vi "Test Bench v12.vi"() -> ()   [LabVIEW 2022 SP3]
uses:
  WhiteNoise.ctl
  <vilib>/Utility/error.llb/DialogType.ctl
  <vilib>/DAQmx/read.llb/DAQmx Read (Analog 1D DBL 1Chan NSamp).vi
  <vilib>/DAQmx/write.llb/DAQmx Write (Analog 2D DBL NChan NSamp).vi
  <vilib>/DAQmx/create/channels.llb/DAQmx Create Channel (AI-Acceleration-Accelerometer).vi
  <vilib>/DAQmx/create/channels.llb/DAQmx Create Channel (AO-Voltage-Basic).vi
  <vilib>/DAQmx/configure/timing.llb/DAQmx Timing (Sample Clock).vi
  <vilib>/DAQmx/miscellaneous.llb/DAQmx Fill In Error Info.vi
  <resource>/objmgr/daqmx.rc
  <vilib>/measure/NI_MABase.lvlib
  <vilib>/DAQmx/configure/task.llb/DAQmx Configure Logging (TDMS).vi
  <vilib>/Waveform/WDTOps.llb/WDT Get Waveform Time Array DBL.vi
panel:
  in  "Folder to save file to":path=path "C:/Users/LAV-UFSC/Documents/LAV-TCC/Dados-Experimentos/Dados-Bancada-LABVIEW"
  in  "Log Raw\nData":bool
  in  "Accel. 2":bool
  in  "Start\nReading":bool=TRUE
  out "New file path":path
  in  "Signal Output Control":enum32{"White Noise", "Harmonic"}(tab)
  in  "White Noise\nParameters":T2={"Seed"=0.0, "Standard Deviation"=0.2, "Reset"=FALSE, "Iterator"=1.0, "Seed"=-1, "Stop 4"=FALSE, "Lower Cut-Off"=5.0, "Upper Cut-Off"=350.0} {"Upper Cut-Off" min=5.0 max=350.0 step=10.0; "Lower Cut-Off" min=5.0 max=350.0 step=10.0; "Standard Deviation" min=0.001 max=1.5 step=0.05 format="%0.2p"}
  in  "Hamonic\nParameters":T3={"Waveform Type"=0, "Frequency"=10.0, "Amplitude"=0.25, "Stop 4"=FALSE} {"Frequency" min=5.0 max=350.0 step=10.0 format="%0.2p"; "Waveform Type" items=["Sine Wave", "Triangle Wave", "Square Wave", "Sawtooth Wave"]; "Amplitude" min=0.001 max=0.3 step=0.05 format="%0.2p"}
  in  "Start\nOutput":bool=TRUE
  # "Filter"
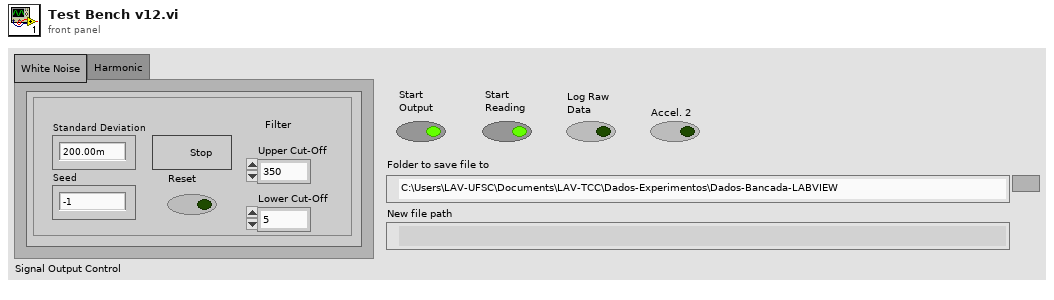
[diagram p1: front panel]
types:
  T1 = typedef "WhiteNoise.ctl" = dbl
  T2 = cluster{"Seed":T1, "Standard Deviation":dbl, "Reset":bool, "Iterator":dbl, "Seed":i8, "Stop 4":bool, "Lower Cut-Off":dbl, "Upper Cut-Off":dbl}
  T3 = cluster{"Waveform Type":u16, "Frequency":dbl, "Amplitude":dbl, "Stop 4":bool}
  T4 = typedef "DialogType.ctl" = u16
  T5 = enum16{"open", "open or create", "create or replace", "create", "open (read-only)"}
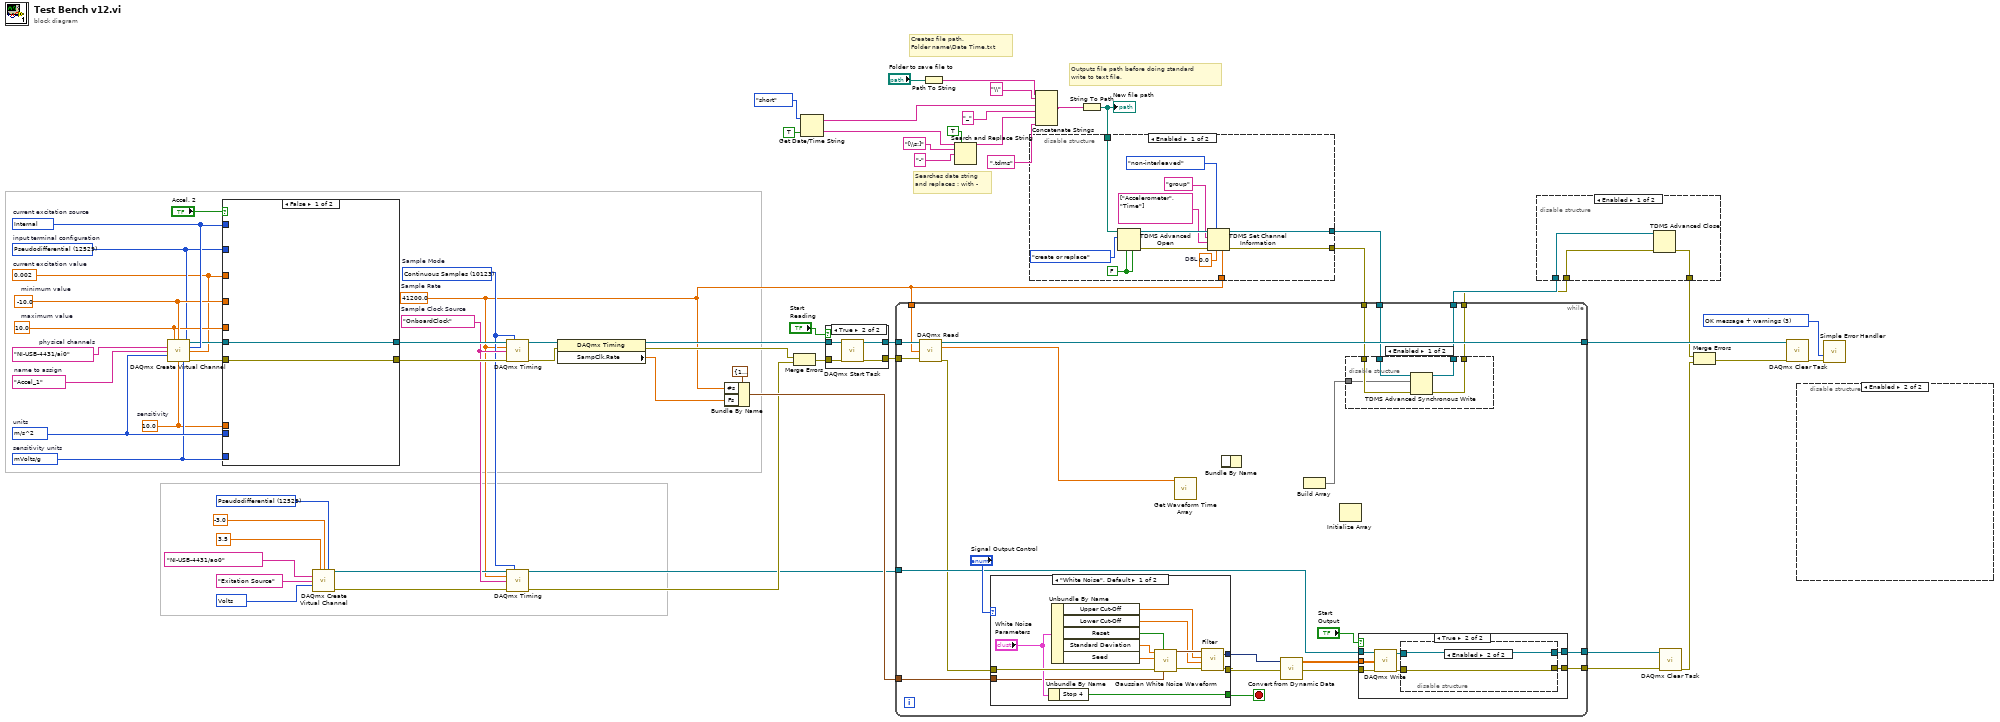
[diagram p0: block diagram]
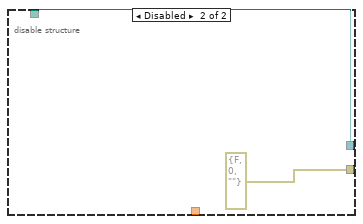
[diagram p2: hidden frame]
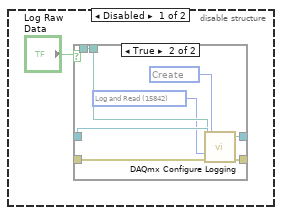
[diagram p4: hidden frame]
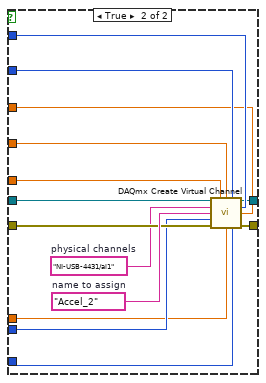
[diagram p6: hidden frame]
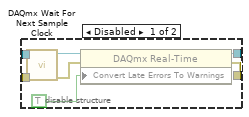
[diagram p10: hidden frame]
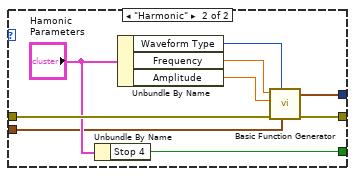
[diagram p11: hidden frame]
diagram:
  w40 = T4 3 items=["no dialog", "OK message", "continue or stop message", "OK message + warnings", "continue/stop + warnings"] ("type of dialog (OK msg:1)")
  w53 = 12529 items=["Default"=-1, "RSE"=10083, "Differential"=10106, "Pseudodifferential"=12529] ("output terminal configuration")
  w51 = 10348 items=["Volts"=10348, "From Custom Scale"=10065] ("units")
  w57 = 12509 items=["mVolts/g"=12509, "Volts/g"=12510]  # sensitivity units
  w44 = 10.0  # sensitivity
  w56 = 0.002  # current excitation value
  w64 = 10200 items=["Internal"=10200, "External"=10167, "None"=10230]  # current excitation source
  w58 = tag "NI-USB-4431/ai0"  # physical channels
  w41 = tag "OnboardClock"  # Sample Clock Source
  w15 = 41200.0  # Sample Rate
  w39 = 10123 items=["Finite Samples"=10178, "Continuous Samples"=10123, "Hardware Timed Single Point"=12522]  # Sample Mode
  w60 = 12529 items=["default"=-1, "RSE"=10083, "NRSE"=10078, "Differential"=10106, "Pseudodifferential"=12529]  # input terminal configuration
  w63 = -10.0  # minimum value
  w62 = 10.0  # maximum value
  w66 = "Accel_1"  # name to assign
  w61 = 12470 items=["g"=10186, "m/s^2"=12470, "in/s^2"=12471, "From Custom Scale"=10065]  # units
  # "Searches date string\nand replaces : with -"
  # "Creates file path.\nFolder name\\Date Time.txt"
  # "Outputs file path before doing standard\nwrite to text file."
  n1 = call-poly <vilib>:"DAQmx Create Virtual Channel.vi"("maximum value"=w62, "minimum value"=w63, "input terminal configuration"=w60, "physical channels"=w58, "current excitation source"=w64, "name to assign"=w66, "current excitation value"=w56, "units"=w61, "sensitivity"=w44, "sensitivity units"=w57) -> ("task out"=w59:refnum<k21>, "error out"=w65:errorcluster)  [unwired: 4 in]
  n2 = case shown="False" "Accel. 2" {
    tunnel: w65 -> [w68 w81]
    tunnel: w64 -> [_ w80]
    tunnel: w63 -> [_ w79]
    tunnel: w62 -> [_ w78]
    tunnel: w61 -> [_ w77]
    tunnel: w60 -> [_ w76]
    tunnel: w59 -> [w67 w75]
    tunnel: w57 -> [_ w73]
    tunnel: w56 -> [_ w72]
    tunnel: w44 -> [_ w71]
    tunnel: [w68 w70] -> w43
    tunnel: [w67 w69] -> w42
    frame False {
    }
    frame True {
      w74 = tag "NI-USB-4431/ai1"  # physical channels
      w82 = "Accel_2"  # name to assign
      n3 = call-poly <vilib>:"DAQmx Create Virtual Channel.vi"("task in"=w75, "maximum value"=w78, "minimum value"=w79, "input terminal configuration"=w76, "physical channels"=w74, "current excitation source"=w80, "name to assign"=w82, "current excitation value"=w72, "units"=w77, "error in"=w81, "sensitivity"=w71, "sensitivity units"=w73) -> ("task out"=w69:refnum<k21>, "error out"=w70:errorcluster)  [unwired: 2 in]
    }
  }
  n4 = call-poly <vilib>:"DAQmx Create Virtual Channel.vi"("maximum value"=3.5, "minimum value"=-3.0, "output terminal configuration"=w53, "physical channels"=tag "NI-USB-4431/ao0", "name to assign"="Exitation Source", "units"=w51) -> ("task out"=w37:refnum<k21>, "error out"=w38:errorcluster)  [unwired: 8 in]
  n5 = call-poly <vilib>:"DAQmx Timing.vi"("task/channels in"=w42, "sample mode"=w39, "rate"=w15, "source"=w41, "error in"=w43) -> ("task out"=w47:refnum<k21>, "error out"=w48:errorcluster)  [unwired: 9 in]
  n6 = call-poly <vilib>:"DAQmx Timing.vi"("task/channels in"=w37, "sample mode"=w39, "rate"=w15, "source"=w41, "error in"=w38) -> ("task out"=w35:refnum<k21>, "error out"=w36:errorcluster)  [unwired: 9 in]
  n7 = property class="DAQmx Timing"(reference=w47, error in=w48) -> (reference out=w31:refnum<k21>, error out=w27:errorcluster, "SampClk.Rate"=w49:dbl)
  n8 = Bundle By Name(cluster=cluster{"Fs":dbl, "#s":dbl} {"Fs"=1000.0, "#s"=1000.0} ("sampling info"), "#s"=w15, "Fs"=w49) -> (w46:cluster{"Fs":dbl, "#s":dbl})
  n9 = Merge Errors(w27, w36) -> (w26:errorcluster)
  n10 = Get Date/Time String(date format (0)=enum16{"short", "long", "abbreviated"}."short", want seconds? (F)=TRUE) -> (date string=w3:string, time string=w12:string)  [unwired: 1 in]
  n11 = case shown="True" "Start\nReading" {
    tunnel: [w83 w85] -> w29
    tunnel: [w84 w86] -> w28
    tunnel: w26 -> [w84 w87]
    tunnel: w31 -> [w83 w88]
    frame False {
    }
    frame True {
      n12 = call <vilib>:"DAQmx Start Task.vi"("task/channels in"=w88, "error in"=w87) -> ("task out"=w85:refnum<k21>, "error out"=w86:errorcluster)  [unwired: 12 in]
    }
  }
  n13 = Path To String(path="Folder to save file to") -> (string=w6:string)
  n14 = Search and Replace String(replace all?=TRUE ("replace all? (F)"), input string=w12, search string="[\\s:]" ("replace string (\"\")"), replace string="-" ("replace string (\"\")")) -> (result string=w4:string)  [unwired: 4 in, 3 out]
  n15 = Concatenate Strings(w6, "\\" ("string"), w3, "_" ("string"), w4, ".tdms" ("string")) -> (w1:string)
  n16 = String To Path(string=w1) -> (path=w23:path)
  "New file path" <- w23
  n17 = disable-structure shown="Enabled" {
    disable-tunnel: w23 -> [w92 w102]
    disable-tunnel: [w91 w102] -> w22
    disable-tunnel: [w90 errorcluster {"status"=FALSE, "code"=0, "source"=""} ("error out")] -> w21
    disable-tunnel: w15 -> [w89 _]
    frame Enabled {
      w93 = 0.0  # DBL
      w95 = FALSE ("enable asynchronous? (T)")
      n18 = TDMS Advanced Open(4:w95, 6:w95, 10:T5."create or replace" ("operation (0:open)"), 11:w92) -> (0:w99:errorcluster, 3:w98:refnum<k34>)  [unwired: 1 in, 1 out]
      n19 = TDMS Set Channel Information(4:w89, 6:w93, 7:enum16{"non-interleaved", "interleaved"}."non-interleaved" ("data layout (0:non-interleaved)"), 8:w99, 9:string[] ["Accelerometer", "Time"] ("channel name(s)"), 10:"group" ("group name (Untitled)"), 11:w98) -> (0:w90:errorcluster, 3:w91:refnum<k34>)
    }
    frame Disabled {
    }
  }
  n20 = while {
    tunnel: w35 -> [w120]
    tunnel: [w114] -> w34
    tunnel: w46 -> [w121]
    tunnel: [w116] -> w33
    tunnel: w29 -> [w119]
    tunnel: w28 -> [w118]
    tunnel: [w115] -> w24
    tunnel: w22 -> [w106]
    tunnel: w21 -> [w111]
    tunnel: [w110] -> w20
    tunnel: [w109] -> w19
    tunnel: w15 -> [w104]
    stop <- w112 stop-if-true
    n21 = call-poly <vilib>:"DAQmx Read.vi"("task/channels in"=w119, "number of samples per channel"=w104, "error in"=w118) -> ("task out"=w115:refnum<k21>, "data"=w103:dbl[], "error out"=w117:errorcluster)  [unwired: 10 in]
    n22 = case shown="\"White Noise\", Default" "Signal Output Control" {
      tunnel: w117 -> [w161 w170]
      tunnel: [w157 w168] -> w122
      tunnel: [w159 w169] -> w108
      tunnel: [w160 w166] -> w112
      tunnel: w121 -> [w154 w165]
      frame "White Noise", Default {
        n23 = Unbundle By Name("White Noise\nParameters") -> ("Stop 4"=w160:bool)
        n24 = Unbundle By Name("White Noise\nParameters") -> ("Upper Cut-Off"=w150:dbl, "Lower Cut-Off"=w149:dbl, "Reset"=w151:bool, "Standard Deviation"=w152:dbl, "Seed"=w153:T1)
        n25 = call <vilib>:"Gaussian White Noise Waveform.vi"("sampling info"=w154, "reset signal"=w151, "error in (no error)"=w161, "seed"=w153, "standard deviation"=w152) -> ("error out"=w158:errorcluster, "signal out"=w155:waveform(dbl))  [unwired: 5 in]
        n26 = call "Filter"("error in (no error)"=w158, "Lower Cut-Off"=w149, "Upper Cut-Off"=w150, "Signal"=w155) -> ("error out"=w157:errorcluster, "Filtered Signal"=w159:dynamicdata)  [unwired: 6 in]
      }
      frame "Harmonic" {
        n27 = Unbundle By Name("Hamonic\nParameters") -> ("Stop 4"=w166:bool)
        n28 = Unbundle By Name("Hamonic\nParameters") -> ("Waveform Type"=w164:u16, "Frequency"=w163:dbl, "Amplitude"=w162:dbl)
        n29 = call <vilib>:"Basic Function Generator.vi"("sampling info"=w165, "signal type"=w164, "error in (no error)"=w170, "amplitude"=w162, "frequency"=w163) -> ("error out"=w168:errorcluster, "signal out"=w169:waveform(dbl))  [unwired: 4 in, 1 out]
      }
    }
    n30 = call-poly <vilib>:"Get Waveform Time Array.vi"("waveform in"=w103) -> ()  [unwired: 9 in, 2 out]
    n31 = Bundle By Name() -> ()  [unwired: 2 in, 1 out]
    n32 = call "Convert from Dynamic Data"("Dynamic Data Type"=w108) -> ("Array"=w113:dbl[][])  [unwired: 3 in]
    n33 = Build Array() -> (w107:void[])  [unwired: 2 in]
    n34 = Initialize Array() -> ()  [unwired: 2 in, 1 out]
    n35 = disable-structure shown="Enabled" {
      disable-tunnel: w111 -> [w128 w130]
      disable-tunnel: [w127 w129] -> w110
      disable-tunnel: [w126 w130] -> w109
      disable-tunnel: w107 -> [w125 _]
      disable-tunnel: w106 -> [w124 w129]
      frame Enabled {
        n36 = TDMS Advanced Synchronous Write(8:w128, 10:w125, 11:w124) -> (0:w126:errorcluster, 3:w127:refnum<k34>)
      }
      frame Disabled {
      }
    }
    n37 = case shown="True" "Start\nOutput" {
      tunnel: w122 -> [w131 w139]
      tunnel: w120 -> [w132 w138]
      tunnel: [w131 w133] -> w116
      tunnel: [w132 w134] -> w114
      tunnel: w113 -> [_ w135]
      frame False {
      }
      frame True {
        n38 = call-poly <vilib>:"DAQmx Write.vi"("task/channels in"=w138, "data"=w135, "error in"=w139) -> ("task out"=w137:refnum<k21>, "error out"=w136:errorcluster)  [unwired: 10 in, 1 out]
        n39 = disable-structure shown="Enabled" {
          disable-tunnel: w137 -> [w146 w147]
          disable-tunnel: w136 -> [w145 w148]
          disable-tunnel: [w143 w147] -> w134
          disable-tunnel: [w142 w148] -> w133
          frame Disabled {
            n40 = call <vilib>:"DAQmx Wait For Next Sample Clock.vi"("task/channels in"=w146, "error in"=w145) -> ("task out"=w144:refnum<k21>, "error out"=w141:errorcluster)  [unwired: 11 in, 1 out]
            n41 = property class="DAQmx Real-Time"(reference=w144, error in=w141, "Convert Late Errors To Warnings"=TRUE ("ConvLateErrorsToWarnings")) -> (reference out=w143:refnum<k21>, error out=w142:errorcluster)
          }
          frame Enabled {
          }
        }
      }
    }
  }
  n42 = disable-structure shown="Enabled" {
    disable-tunnel: w20 -> [w173 _]
    disable-tunnel: w19 -> [w172 w174]
    disable-tunnel: [w171 w174] -> w16
    frame Enabled {
      n43 = TDMS Advanced Close(8:w172, 11:w173) -> (0:w171:errorcluster)  [unwired: 2 in, 1 out]
    }
    frame Disabled {
    }
  }
  n44 = call <vilib>:"DAQmx Clear Task.vi"("task in"=w34, "error in"=w33) -> ("error out"=w17:errorcluster)  [unwired: 13 in]
  n45 = Merge Errors(w16, w17) -> (w18:errorcluster)
  n46 = call <vilib>:"DAQmx Clear Task.vi"("task in"=w24, "error in"=w18) -> ("error out"=w25:errorcluster)  [unwired: 13 in]
  n47 = disable-structure shown="Enabled" {
    frame Disabled {
      n48 = case shown="True" "Log Raw\nData" {
        tunnel: _ -> [w177 w184]
        tunnel: [w177 w183] -> _
        tunnel: _ -> [_ w181]
        tunnel: [_ w181] -> _
        tunnel: _ -> [w176 w179]
        tunnel: [w176 w180] -> _
        frame False {
        }
        frame True {
          w182 = 15848 items=["Open"=10437, "Open or Create"=15846, "Create or Replace"=15847, "Create"=15848] ("operation")
          w178 = 15842 items=["Off"=10231, "Log"=15844, "Log and Read"=15842] ("logging mode")
          n49 = call-poly <vilib>:"DAQmx Configure Logging.vi"("task/channels in"=w184, "operation"=w182, "file path"=w181, "logging mode"=w178, "error in"=w179) -> ("task out"=w183:refnum<k21>, "error out"=w180:errorcluster)  [unwired: 9 in]
        }
      }
    }
    frame Enabled {
    }
  }
  n50 = call <vilib>:"Simple Error Handler.vi"("type of dialog (OK msg:1)"=w40, "error in (no error)"=w25) -> ()  [unwired: 3 in, 5 out]
